vi "ConstellationParseBoard.vi"(8 "error in":errorcluster, 11 "String":string) -> (0 "error out":errorcluster, 1 "Temperature":sgl, 2 "Status":i8[](array[numeric]), 3 "Bchip":sgl[][](array[numeric]))   [LabVIEW 2012]
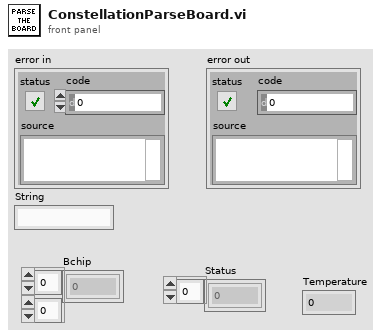
[diagram p1: front panel]
types:
  T1 = enum16{"big-endian, network order", "native, host order", "little-endian"}
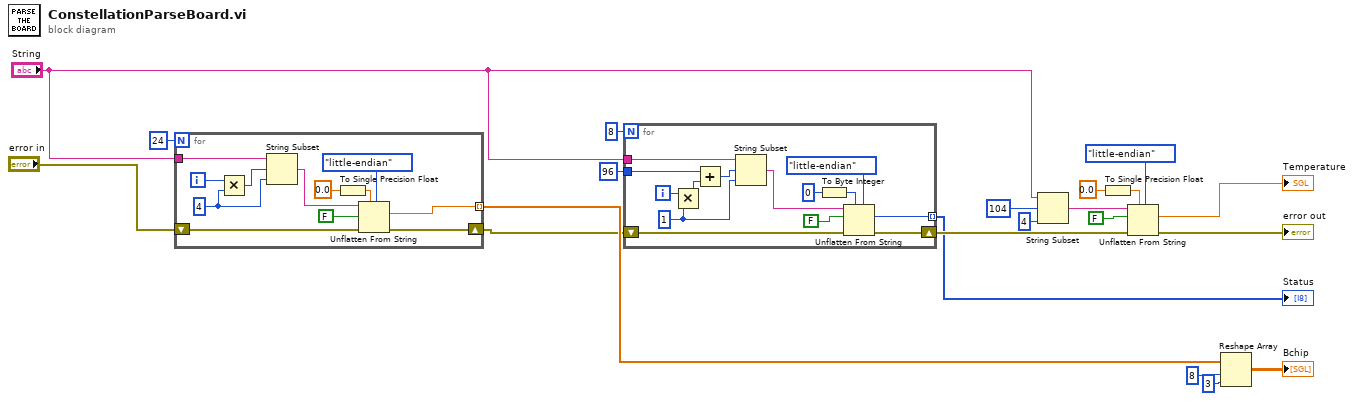
[diagram p0: block diagram]
diagram:
  n1 = for {
    N: 24 -> [_]
    tunnel: [w27] -> w20 mode=indexing
    tunnel: "String" -> [w24]
    shift-right: [w22] -> w14
    shift-left: "error in" -> [w23]
    i -> [w33]
    w25 = 4 ("y")
    n2 = Multiply(x=w33, y=w25) -> (x*y=w26:i32)
    n3 = String Subset(string=w24, offset (0)=w26, length (rest)=w25) -> (substring=w28:string)
    n4 = To Single Precision Float(number=0.0) -> (single precision float=w29:sgl)
    n5 = Unflatten From String(type=w29, binary string=w28, data includes array or string size? (T)=FALSE, byte order (0:big-endian, network order)=T1."little-endian", error in (no error)=w23) -> (value=w27:sgl, error out=w22:errorcluster)  [unwired: 1 out]
  }
  n6 = for {
    N: 8 -> [_]
    tunnel: "String" -> [w47]
    tunnel: [w42] -> w4 mode=indexing
    tunnel: 96 -> [w36]
    shift-right: [w34] -> w15
    shift-left: w14 -> [w35]
    i -> [w46]
    w41 = 1 ("y")
    n7 = Multiply(x=w46, y=w41) -> (x*y=w38:i32)
    n8 = Add(x=w36, y=w38) -> (x+y=w37:i32)
    n9 = String Subset(string=w47, offset (0)=w37, length (rest)=w41) -> (substring=w43:string)
    n10 = To Byte Integer(number=i8 0) -> (8bit integer=w40:i8)
    n11 = Unflatten From String(type=w40, binary string=w43, data includes array or string size? (T)=FALSE, byte order (0:big-endian, network order)=T1."little-endian", error in (no error)=w35) -> (value=w42:i8, error out=w34:errorcluster)  [unwired: 1 out]
  }
  "Status" <- w4
  n12 = String Subset(string="String", offset (0)=104, length (rest)=4 ("y")) -> (substring=w10:string)
  n13 = To Single Precision Float(number=0.0) -> (single precision float=w7:sgl)
  n14 = Unflatten From String(type=w7, binary string=w10, data includes array or string size? (T)=FALSE, byte order (0:big-endian, network order)=T1."little-endian", error in (no error)=w15) -> (value=→"Temperature":sgl, error out=→"error out":errorcluster)  [unwired: 1 out]
  n15 = Reshape Array(w20, 8 ("dimension size"), 3 ("dimension size")) -> (→"Bchip":sgl[][])
